vi "Analyze Read.vi"(0 "VISA in":refnum<visa-resource-name>, 1 "String":string, 3 "error in (no error)":errorcluster) -> (7 "VISA out":refnum<visa-resource-name>, 8 "Stop?":bool, 10 "error out":errorcluster)   [LabVIEW 2017]
panel:
  out "VIN":u32
  out "LWST":u32
  out "EDGA":u32
  out "SPMB":u32
  out "SPMA":u32
  out "LED2":u32
  out "STAT":u32 format="%.0x"
  out "FCT":u32
  out "STEP":u32
  out "SPM":u32
  out "CLR":u32
  out "MAMP":u32
  out "Prta Number":string
  out "Prts Number":string
  out "BLD":u32
  out "EE ROM":string
  out "Array Size":i32
  out "Part Number":string
  out "VBUS":u32
  out "EERD":u32 format="%.0x"
  out "LOOP":u32 format="%.0x"
  out "LFTG":u32
  out "LFTS":u32
  out "LIFT":u32
  out "BRK":u32
  out "RPMH":u32
  out "RPML":u32
  out "PRPM":u32
  out "REV":u32
  out "RPM":u32
  out "SECS":u32
  out "ACAD":u32
  out "BATL":u32
  out "BATC":u32
  out "VCHG":u32
  out "VBAT":u32
  out "RES":u32
  out "RAMP":u32
  out "Error Codes":u8[](array[numeric])
  out "Array":string[](array[string])
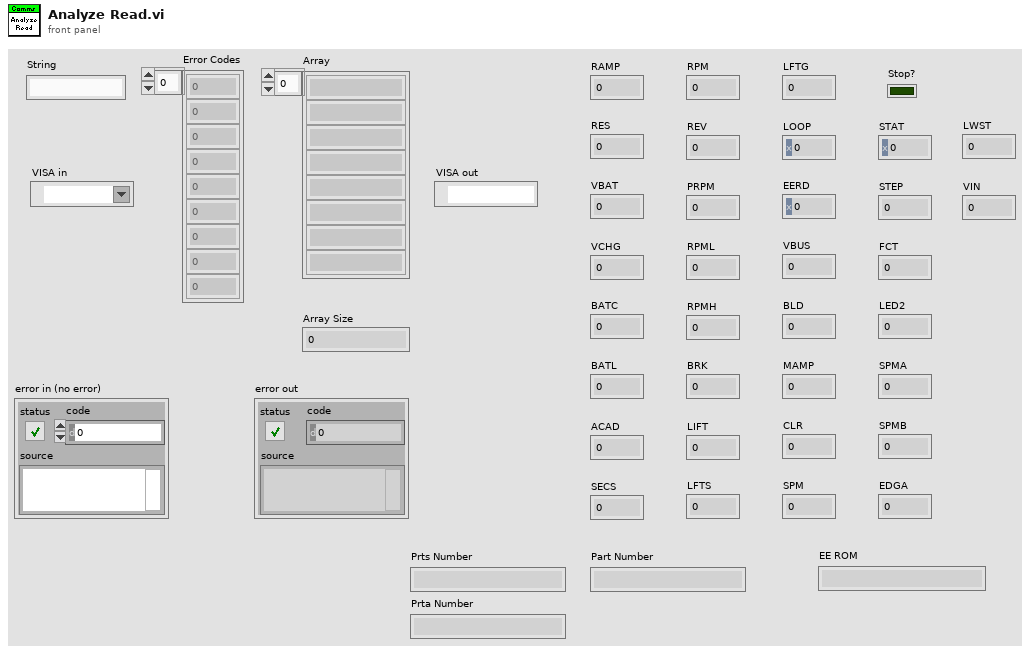
[diagram p1: front panel]
types:
  T1 = enum16{"Init", "Get Index", "Analyze Part", "Analyze Prts", "Analyze Prta", "Set VER", "Set TYPE"}
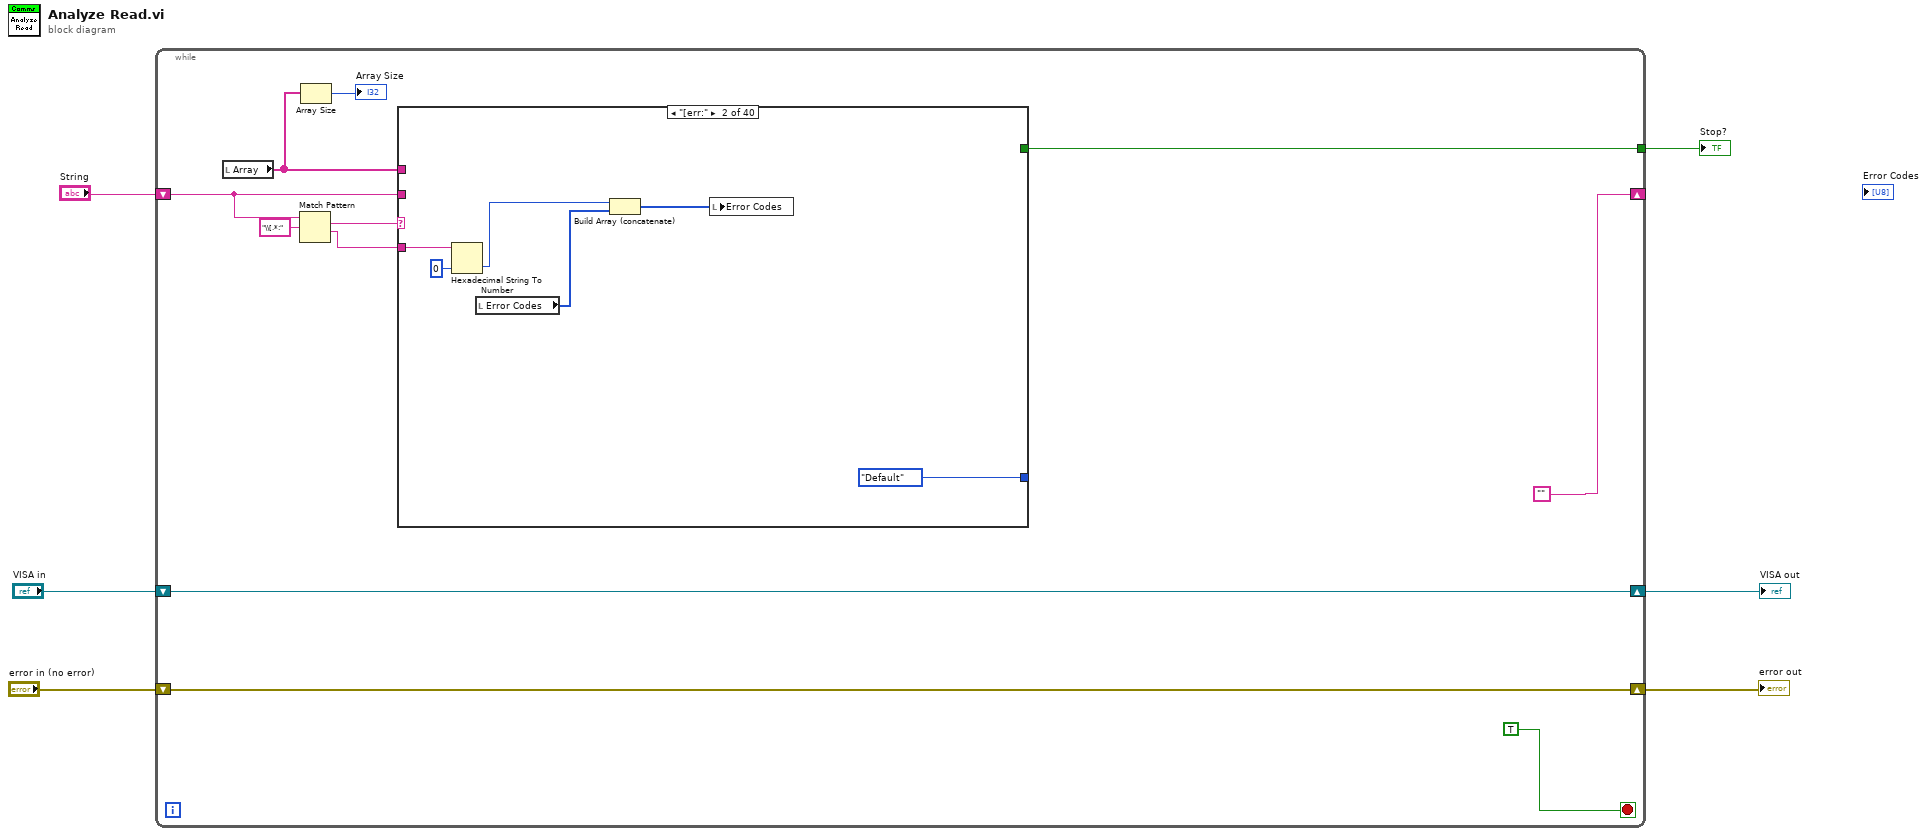
[diagram p0: block diagram]
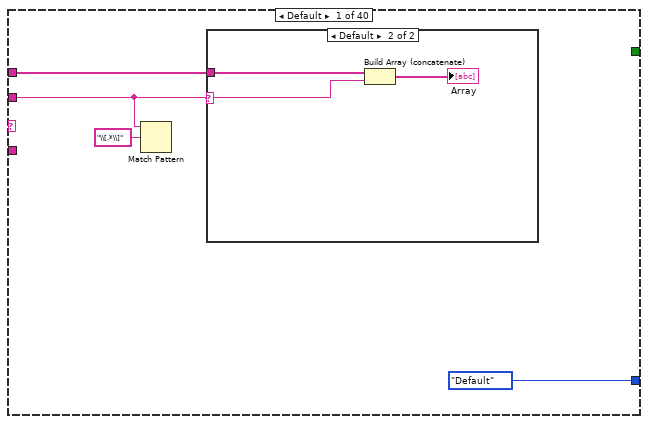
[diagram p2: hidden frame]
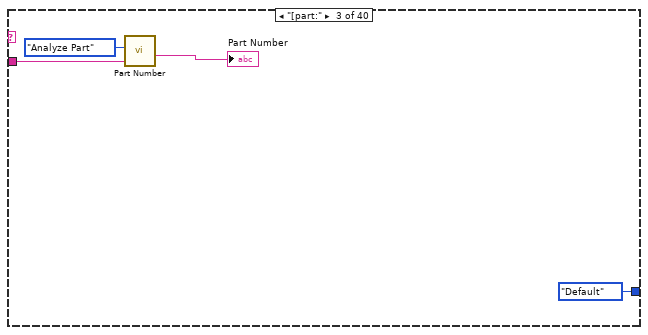
[diagram p4: hidden frame]
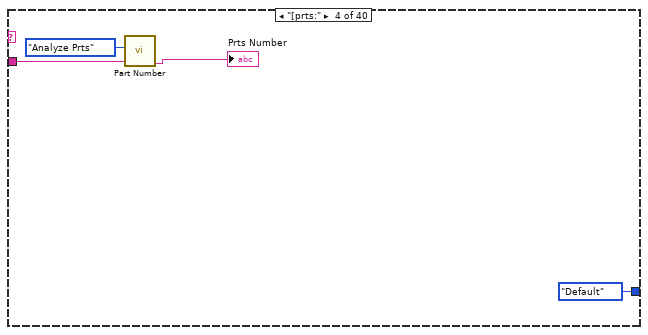
[diagram p5: hidden frame]
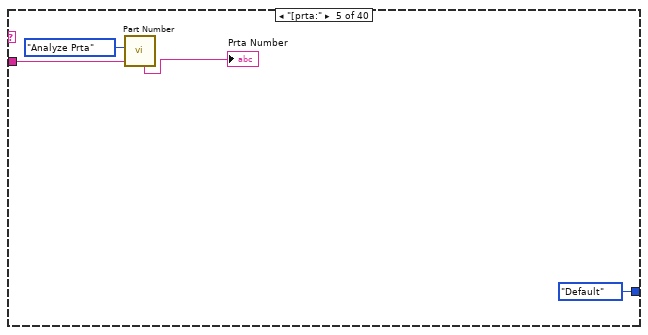
[diagram p6: hidden frame]
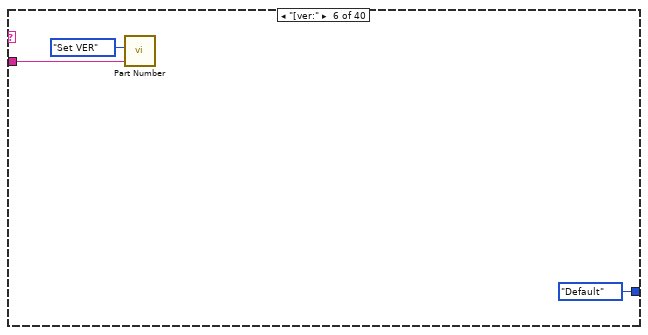
[diagram p7: hidden frame]
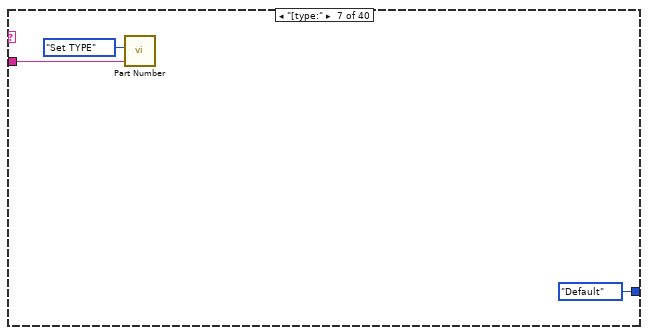
[diagram p8: hidden frame]
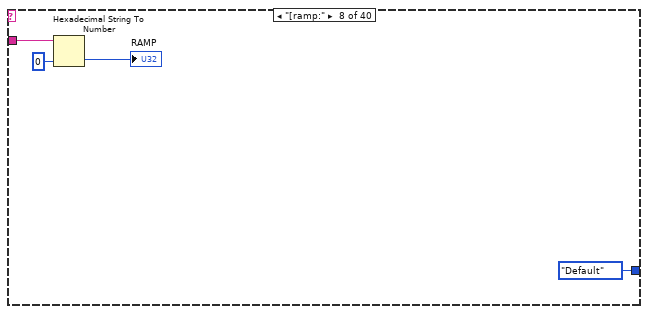
[diagram p9: hidden frame]
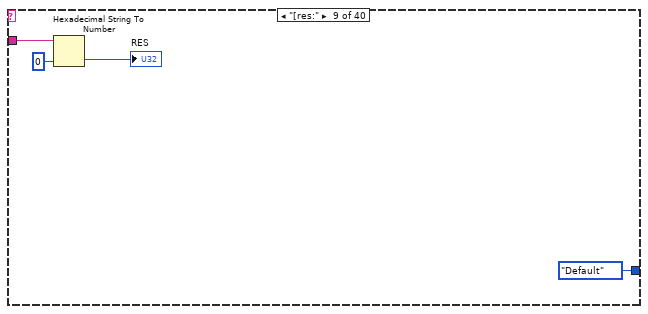
[diagram p10: hidden frame]
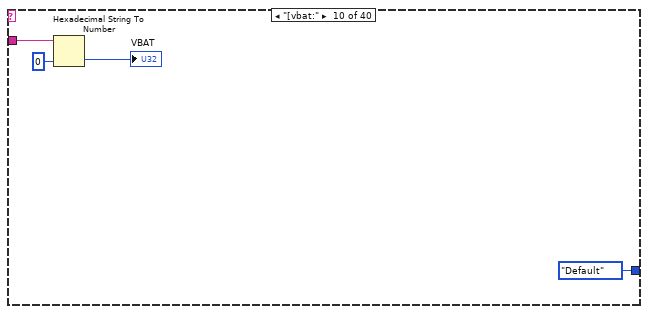
[diagram p11: hidden frame]
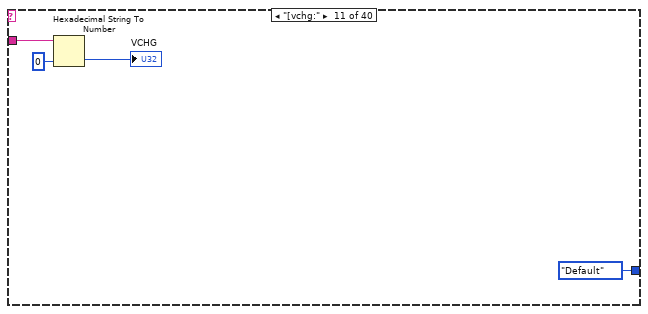
[diagram p12: hidden frame]
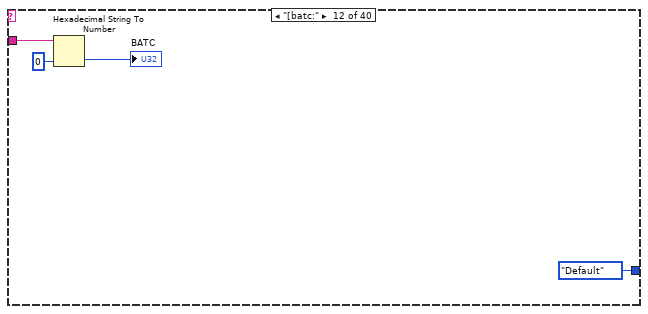
[diagram p13: hidden frame]
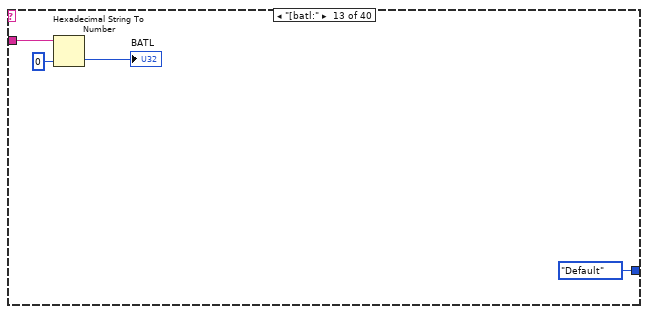
[diagram p14: hidden frame]
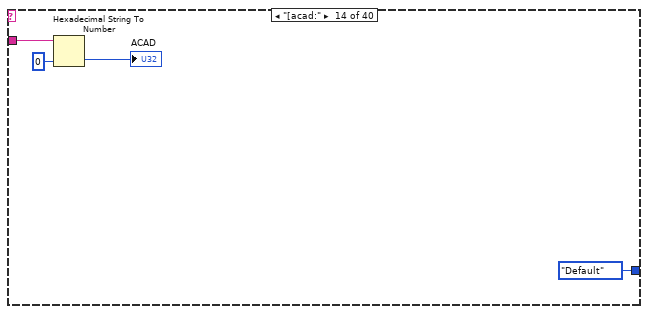
[diagram p15: hidden frame]
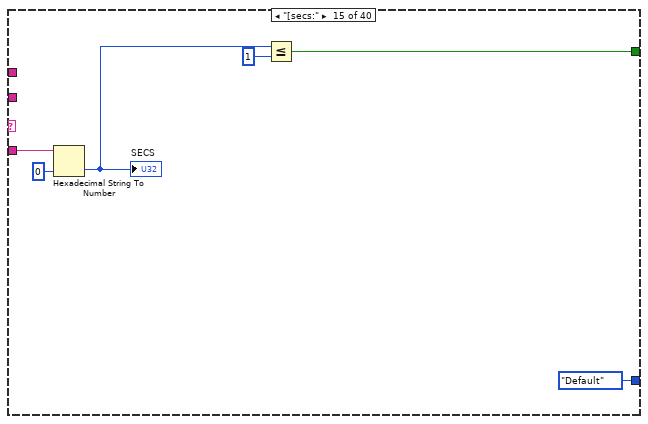
[diagram p16: hidden frame]
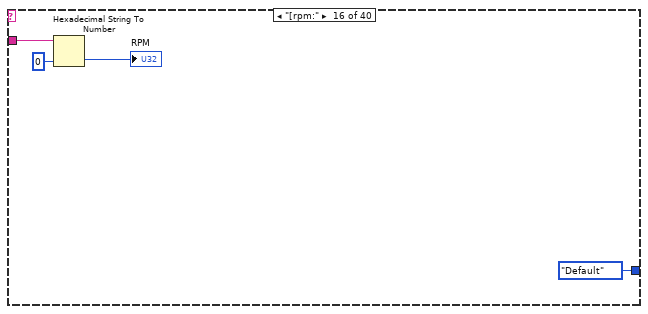
[diagram p17: hidden frame]
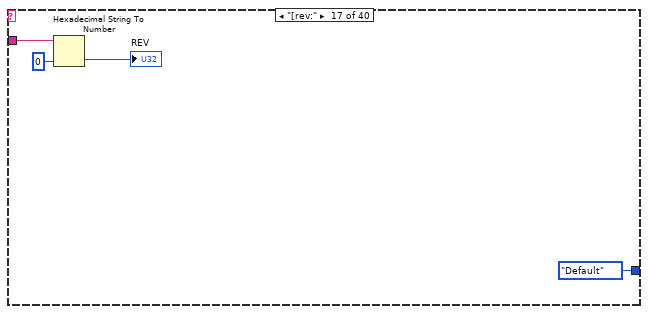
[diagram p18: hidden frame]
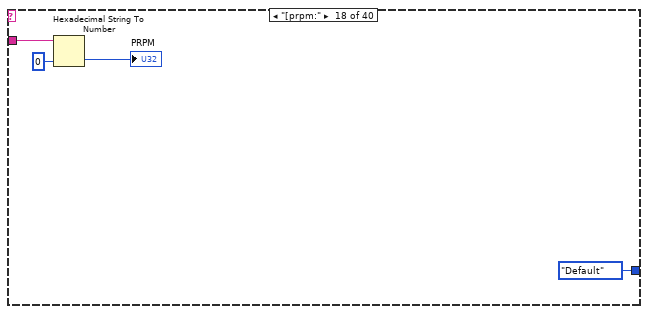
[diagram p19: hidden frame]
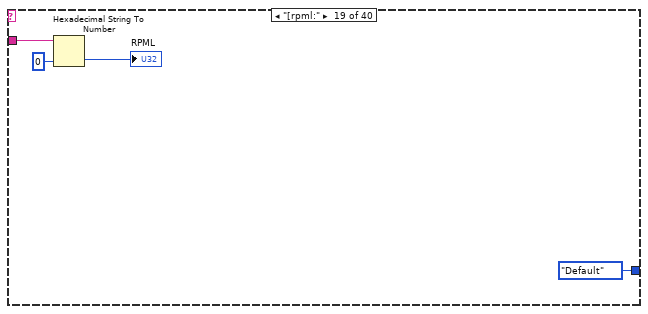
[diagram p20: hidden frame]
diagram:
  n1 = while {
    shift-right: [w13] -> w3
    shift-left: "VISA in" -> [w13]
    shift-right: [w12] -> w2
    shift-left: "error in (no error)" -> [w12]
    shift-right: [""] -> _
    shift-left: "String" -> [w14]
    tunnel: [w7] -> w1
    stop <- TRUE stop-if-true
    n2 = local read "Array"() -> (w8:string[])
    n3 = Match Pattern(string=w14, regular expression="\\[.*:") -> (match substring=w16:string, after substring=w15:string)  [unwired: 1 in, 2 out]
    n4 = Array Size(array=w8) -> (size(s)=→"Array Size":i32)
    n5 = case shown="\"[err:\"" w16 {
      tunnel: w15 -> [_ w29 w33 w37 w41 w44 w47 w51 w55 w59 w63 w67 w71 w75 w81 w85 w89 w93 w97 w101 w105 w109 w113 w117 w121 w125 w131 w135 w139 w143 w147 w151 w155 w159 w163 w167 w171 w175 w179 w183]
      tunnel: w14 -> [w19 _ _ _ _ _ _ _ _ _ _ _ _ _ _ _ _ _ _ _ _ _ _ _ _ _ _ _ _ _ _ _ _ _ _ _ _ _ _ _]
      tunnel: [enum16{"Default", "Send RSET"}."Default" enum16{"Default", "Send RSET"}."Default" enum16{"Default", "Send RSET"}."Default" enum16{"Default", "Send RSET"}."Default" enum16{"Default", "Send RSET"}."Default" enum16{"Default", "Send RSET"}."Default" enum16{"Default", "Send RSET"}."Default" enum16{"Default", "Send RSET"}."Default" enum16{"Default", "Send RSET"}."Default" enum16{"Default", "Send RSET"}."Default" enum16{"Default", "Send RSET"}."Default" enum16{"Default", "Send RSET"}."Default" enum16{"Default", "Send RSET"}."Default" enum16{"Default", "Send RSET"}."Default" enum16{"Default", "Send RSET"}."Default" enum16{"Default", "Send RSET"}."Default" enum16{"Default", "Send RSET"}."Default" enum16{"Default", "Send RSET"}."Default" enum16{"Default", "Send RSET"}."Default" enum16{"Default", "Send RSET"}."Default" enum16{"Default", "Send RSET"}."Default" enum16{"Default", "Send RSET"}."Default" enum16{"Default", "Send RSET"}."Default" enum16{"Default", "Send RSET"}."Default" enum16{"Default", "Send RSET"}."Default" enum16{"Default", "Send RSET"}."Default" enum16{"Default", "Send RSET"}."Default" enum16{"Default", "Send RSET"}."Default" enum16{"Default", "Send RSET"}."Default" enum16{"Default", "Send RSET"}."Default" enum16{"Default", "Send RSET"}."Default" enum16{"Default", "Send RSET"}."Default" enum16{"Default", "Send RSET"}."Default" enum16{"Default", "Send RSET"}."Default" enum16{"Default", "Send RSET"}."Default" enum16{"Default", "Send RSET"}."Default" enum16{"Default", "Send RSET"}."Default" enum16{"Default", "Send RSET"}."Default" enum16{"Default", "Send RSET"}."Default" enum16{"Default", "Send RSET"}."Default"] -> _
      tunnel: w8 -> [w18 _ _ _ _ _ _ _ _ _ _ _ _ _ _ _ _ _ _ _ _ _ _ _ _ _ _ _ _ _ _ _ _ _ _ _ _ _ _ _]
      tunnel: [_ _ _ _ _ _ _ _ _ _ _ _ _ _ w77 _ _ _ _ _ _ _ _ _ _ _ _ _ _ _ _ _ _ _ _ _ _ _ _ _] -> w7
      frame Default {
        n6 = Match Pattern(string=w19, regular expression="\\[.*\\]") -> ()  [unwired: 1 in, 4 out]
        n7 = case shown="Default" w19 {
          selector: w19 -> [_ w24]
          tunnel: w18 -> [_ w23]
          frame "[err]" {
          }
          frame Default {
            n8 = Build Array (concatenate)(w23, w24) -> (→"Array":string[])
          }
        }
      }
      frame "[err:" {
        n9 = Hexadecimal String To Number(string=w29, default (0uL)=u8 0 ("default (0 U32)")) -> (number=w25:u8)  [unwired: 1 in, 1 out]
        n10 = local read "Error Codes"() -> (w28:u8[])
        n11 = Build Array (concatenate)(w25, w28) -> (w27:u8[])
        n12 = local write "Error Codes"(w27) -> ()
      }
      frame "[part:" {
        n13 = call "Part Number.vi"("Value from LPCA"=w33, "Command"=T1."Analyze Part") -> ("Part Number"=→"Part Number":string)  [unwired: 4 in, 5 out]
      }
      frame "[prts:" {
        n14 = call "Part Number.vi"("Value from LPCA"=w37, "Command"=T1."Analyze Prts") -> ("Prts Number"=→"Prts Number":string)  [unwired: 4 in, 5 out]
      }
      frame "[prta:" {
        n15 = call "Part Number.vi"("Value from LPCA"=w41, "Command"=T1."Analyze Prta") -> ("Prta Number"=→"Prta Number":string)  [unwired: 4 in, 5 out]
      }
      frame "[ver:" {
        n16 = call "Part Number.vi"("Value from LPCA"=w44, "Command"=T1."Set VER") -> ()  [unwired: 4 in, 6 out]
      }
      frame "[type:" {
        n17 = call "Part Number.vi"("Value from LPCA"=w47, "Command"=T1."Set TYPE") -> ()  [unwired: 4 in, 6 out]
      }
      frame "[ramp:" {
        n18 = Hexadecimal String To Number(string=w51, default (0uL)=u32 0 ("default (0 U32)")) -> (number=→"RAMP":u32)  [unwired: 1 in, 1 out]
      }
      frame "[res:" {
        n19 = Hexadecimal String To Number(string=w55, default (0uL)=u32 0 ("default (0 U32)")) -> (number=→"RES":u32)  [unwired: 1 in, 1 out]
      }
      frame "[vbat:" {
        n20 = Hexadecimal String To Number(string=w59, default (0uL)=u32 0 ("default (0 U32)")) -> (number=→"VBAT":u32)  [unwired: 1 in, 1 out]
      }
      frame "[vchg:" {
        n21 = Hexadecimal String To Number(string=w63, default (0uL)=u32 0 ("default (0 U32)")) -> (number=→"VCHG":u32)  [unwired: 1 in, 1 out]
      }
      frame "[batc:" {
        n22 = Hexadecimal String To Number(string=w67, default (0uL)=u32 0 ("default (0 U32)")) -> (number=→"BATC":u32)  [unwired: 1 in, 1 out]
      }
      frame "[batl:" {
        n23 = Hexadecimal String To Number(string=w71, default (0uL)=u32 0 ("default (0 U32)")) -> (number=→"BATL":u32)  [unwired: 1 in, 1 out]
      }
      frame "[acad:" {
        n24 = Hexadecimal String To Number(string=w75, default (0uL)=u32 0 ("default (0 U32)")) -> (number=→"ACAD":u32)  [unwired: 1 in, 1 out]
      }
      frame "[secs:" {
        n25 = Hexadecimal String To Number(string=w81, default (0uL)=u32 0 ("default (0 U32)")) -> (number=w79:u32)  [unwired: 1 in, 1 out]
        "SECS" <- w79
        n26 = Less Or Equal?(x=w79, y=u32 1) -> (x <= y?=w77:bool)
      }
      frame "[rpm:" {
        n27 = Hexadecimal String To Number(string=w85, default (0uL)=u32 0 ("default (0 U32)")) -> (number=→"RPM":u32)  [unwired: 1 in, 1 out]
      }
      frame "[rev:" {
        n28 = Hexadecimal String To Number(string=w89, default (0uL)=u32 0 ("default (0 U32)")) -> (number=→"REV":u32)  [unwired: 1 in, 1 out]
      }
      frame "[prpm:" {
        n29 = Hexadecimal String To Number(string=w93, default (0uL)=u32 0 ("default (0 U32)")) -> (number=→"PRPM":u32)  [unwired: 1 in, 1 out]
      }
      frame "[rpml:" {
        n30 = Hexadecimal String To Number(string=w97, default (0uL)=u32 0 ("default (0 U32)")) -> (number=→"RPML":u32)  [unwired: 1 in, 1 out]
      }
      frame "[rpmh:" {
        n31 = Hexadecimal String To Number(string=w101, default (0uL)=u32 0 ("default (0 U32)")) -> (number=→"RPMH":u32)  [unwired: 1 in, 1 out]
      }
      frame "[brk:" {
        n32 = Hexadecimal String To Number(string=w105, default (0uL)=u32 0 ("default (0 U32)")) -> (number=→"BRK":u32)  [unwired: 1 in, 1 out]
      }
      frame "[lift:" {
        n33 = Hexadecimal String To Number(string=w109, default (0uL)=u32 0 ("default (0 U32)")) -> (number=→"LIFT":u32)  [unwired: 1 in, 1 out]
      }
      frame "[lfts:" {
        n34 = Hexadecimal String To Number(string=w113, default (0uL)=u32 0 ("default (0 U32)")) -> (number=→"LFTS":u32)  [unwired: 1 in, 1 out]
      }
      frame "[lftg:" {
        n35 = Hexadecimal String To Number(string=w117, default (0uL)=u32 0 ("default (0 U32)")) -> (number=→"LFTG":u32)  [unwired: 1 in, 1 out]
      }
      frame "[loop:" {
        n36 = Hexadecimal String To Number(string=w121, default (0uL)=u32 0 ("default (0 U32)")) -> (number=→"LOOP":u32)  [unwired: 1 in, 1 out]
      }
      frame "[eerd:" {
        n37 = Hexadecimal String To Number(string=w125, default (0uL)=u32 0 ("default (0 U32)")) -> (number=→"EERD":u32)  [unwired: 1 in, 1 out]
        n38 = call "ROM Data.vi"("Value from LPCA"=w125, "Command"=enum16{"Init", "Get Index", "Analyze"}."Analyze") -> ("ROM Data"=→"EE ROM":string)  [unwired: 1 out]
      }
      frame "[vbus:" {
        n39 = Hexadecimal String To Number(string=w131, default (0uL)=u32 0 ("default (0 U32)")) -> (number=→"VBUS":u32)  [unwired: 1 in, 1 out]
      }
      frame "[vin:" {
        n40 = Hexadecimal String To Number(string=w135, default (0uL)=u32 0 ("default (0 U32)")) -> (number=→"VIN":u32)  [unwired: 1 in, 1 out]
      }
      frame "[bld:" {
        n41 = Hexadecimal String To Number(string=w139, default (0uL)=u32 0 ("default (0 U32)")) -> (number=→"BLD":u32)  [unwired: 1 in, 1 out]
      }
      frame "[mamp:" {
        n42 = Hexadecimal String To Number(string=w143, default (0uL)=u32 0 ("default (0 U32)")) -> (number=→"MAMP":u32)  [unwired: 1 in, 1 out]
      }
      frame "[clr:" {
        n43 = Hexadecimal String To Number(string=w147, default (0uL)=u32 0 ("default (0 U32)")) -> (number=→"CLR":u32)  [unwired: 1 in, 1 out]
      }
      frame "[spm:" {
        n44 = Hexadecimal String To Number(string=w151, default (0uL)=u32 0 ("default (0 U32)")) -> (number=→"SPM":u32)  [unwired: 1 in, 1 out]
      }
      frame "[step:" {
        n45 = Hexadecimal String To Number(string=w155, default (0uL)=u32 0 ("default (0 U32)")) -> (number=→"STEP":u32)  [unwired: 1 in, 1 out]
      }
      frame "[stat:" {
        n46 = Hexadecimal String To Number(string=w159, default (0uL)=u32 0 ("default (0 U32)")) -> (number=→"STAT":u32)  [unwired: 1 in, 1 out]
      }
      frame "[fct:" {
        n47 = Hexadecimal String To Number(string=w163, default (0uL)=u32 0 ("default (0 U32)")) -> (number=→"FCT":u32)  [unwired: 1 in, 1 out]
      }
      frame "[led2:" {
        n48 = Hexadecimal String To Number(string=w167, default (0uL)=u32 0 ("default (0 U32)")) -> (number=→"LED2":u32)  [unwired: 1 in, 1 out]
      }
      frame "[spma:" {
        n49 = Hexadecimal String To Number(string=w171, default (0uL)=u32 0 ("default (0 U32)")) -> (number=→"SPMA":u32)  [unwired: 1 in, 1 out]
      }
      frame "[spmb:" {
        n50 = Hexadecimal String To Number(string=w175, default (0uL)=u32 0 ("default (0 U32)")) -> (number=→"SPMB":u32)  [unwired: 1 in, 1 out]
      }
      frame "[edga:" {
        n51 = Hexadecimal String To Number(string=w179, default (0uL)=u32 0 ("default (0 U32)")) -> (number=→"EDGA":u32)  [unwired: 1 in, 1 out]
      }
      frame "[lwst:" {
        n52 = Hexadecimal String To Number(string=w183, default (0uL)=u32 0 ("default (0 U32)")) -> (number=→"LWST":u32)  [unwired: 1 in, 1 out]
      }
    }
  }
  "error out" <- w2
  "VISA out" <- w3
  "Stop?" <- w1
